vi "VLine.vi"(4 "Properties":T1={"Line"={"Style"=enum."Automatic", "Color"=2147483647, "Width"=nan}, "Display"={"Alpha"=nan, "Z Order"=nan}} {"Line"."Color" items=["Automatic"=2147483647, "Black"=0, "White"=16777215, "Red"=16711680, "Green"=2263842, "Blue"=255, "Cyan"=65535, "Magenta"=16711935, "Yellow"=16776960]}, 5 "Y Max (plot coords)":dbl=nan, 7 "Y Min (plot coords)":dbl=nan, 8 "error in (no error)":errorcluster, 10 "X (data coords)":dbl, 11 "Plot ID":T6 format="%x") -> (0 "error out":errorcluster, 3 "Plot ID Out":T6 format="%x")   [LabVIEW 2013, in "Advanced Plotting Toolkit.lvlib"]
doc: "Display a vertical line on the plot, centered at a particular X location."
uses:
  Advanced Plotting Toolkit.lvlib
  typedefs/PlotID.ctl
  HVLineProperties.ctl
  properties/Line.ctl
  properties/Line_Style.ctl
  typedefs/PlotColor.ctl
  properties/Display.ctl
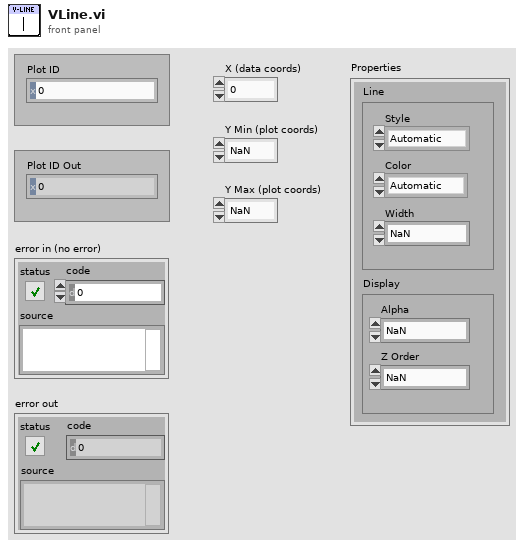
[diagram p1: front panel]
types:
  T1 = typedef "Advanced Plotting Toolkit.lvlib/HVLineProperties.ctl" = cluster{"Line":T2, "Display":T5}
  T2 = typedef "Advanced Plotting Toolkit.lvlib/Line.ctl" = cluster{"Style":T3, "Color":T4, "Width":sgl}
  T3 = typedef "Advanced Plotting Toolkit.lvlib/Line_Style.ctl" = enum16{"Automatic", "Solid", "Dashed", "Dotted", "Dash-dot", "Invisible"}
  T4 = typedef "Advanced Plotting Toolkit.lvlib/PlotColor.ctl" = u32
  T5 = typedef "Advanced Plotting Toolkit.lvlib/Display.ctl" = cluster{"Alpha":dbl, "Z Order":dbl}
  T6 = typedef "Advanced Plotting Toolkit.lvlib/PlotID.ctl" = i32
  T7 = typedef "Advanced Plotting Toolkit.lvlib/KeyValue.ctl" = cluster{"Key":string, "Value":string}
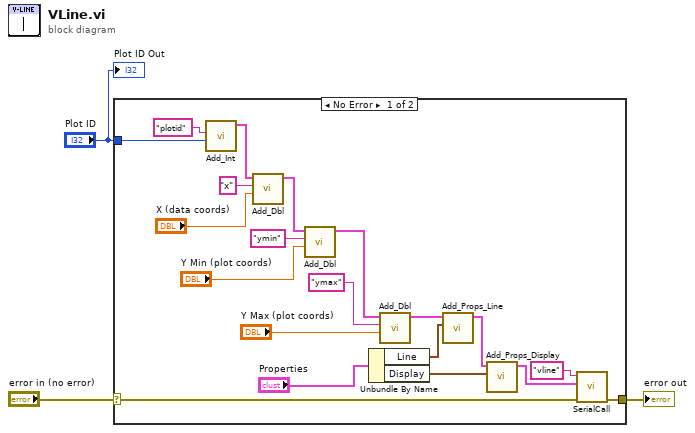
[diagram p0: block diagram]
diagram:
  n1 = case shown="No Error" "error in (no error)" {
    selector: "error in (no error)" -> [w10 w24]
    tunnel: "Plot ID" -> [w14 _]
    tunnel: [w9 w24] -> w1
    frame No Error {
      n2 = call "Add_Int.vi"("Value"=w14, "Key"="plotid") -> ("Keyword Array Out"=w15:T7[])  [unwired: 9 in]
      n3 = call "Add_Dbl.vi"("Value"="X (data coords)", "Key"="x", "Keyword Array"=w15) -> ("Keyword Array Out"=w20:T7[])  [unwired: 8 in]
      n4 = call "Add_Dbl.vi"("Value"="Y Min (plot coords)", "Key"="ymin", "Keyword Array"=w20) -> ("Keyword Array Out"=w19:T7[])  [unwired: 8 in]
      n5 = Unbundle By Name("Properties") -> ("Line"=w8:T2, "Display"=w6:T5)
      n6 = call "Add_Dbl.vi"("Value"="Y Max (plot coords)", "Key"="ymax", "Keyword Array"=w19) -> ("Keyword Array Out"=w18:T7[])  [unwired: 8 in]
      n7 = call "Add_Props_Line.vi"("Line"=w8, "Keyword Array"=w18) -> ("Keyword Array Out"=w5:T7[])  [unwired: 9 in]
      n8 = call "Add_Props_Display.vi"("Display"=w6, "Keyword Array"=w5) -> ("Keyword Array Out"=w4:T7[])  [unwired: 9 in]
      n9 = call "SerialCall.vi"("error in (no error)"=w10, "data"=w4, "Resource"="vline") -> ("error out"=w9:errorcluster)  [unwired: 7 in, 1 out]
    }
    frame Error {
    }
  }
  "error out" <- w1
  "Plot ID Out" <- "Plot ID"
